vi "VALEW_ATC_Verify Concurrent.vi"(0 "GEA2 Reference In":refnum<k24>, 11 "Error In":errorcluster) -> (4 "GEA2 Reference Out":refnum<k24>, 6 "Pass/fail?":bool, 8 "Report Text":string, 15 "Error Out":errorcluster)   [LabVIEW 2016, in "TLMB.lvlib"]
doc: "This test covers the ATC algorithm when doing a concurrent fill. A concurrent fill allows both hot and cold valves to be on at the same time. The valves are operated in parallel."
uses:
  Projects/TLMB.lvlib
  Q:/Common/DLLs/GEA3/GeaCommunication.dll
  Common/DLLs/GEA3/GeaCommunication.dll
  Common/LabVIEW GEA2 Toolkit/LabVIEW_GEA2_Toolkit.lvlibp/type defs/Source_Destination.ctl
  TLMB Common/type defs/MC_Cycle_Engine_Request_State.ctl
  Common/LabVIEW GEA2 Toolkit/LabVIEW_GEA2_Toolkit.lvlibp/type defs/ERD Write Data In.ctl
  Common/LabVIEW GEA2 Toolkit/LabVIEW_GEA2_Toolkit.lvlibp/type defs/Data Type.ctl
  Common/LabVIEW GEA2 Toolkit/LabVIEW_GEA2_Toolkit.lvlibp/type defs/ERD Read Data In.ctl
  <vilib>/DAQmx/write.llb/DAQmx Write (Analog DBL 1Chan 1Samp).vi
  <vilib>/DAQmx/create/channels.llb/DAQmx Create Channel (AO-Voltage-Basic).vi
  <vilib>/DAQmx/miscellaneous.llb/DAQmx Fill In Error Info.vi
  Common/LabVIEW GEA2 Toolkit/LabVIEW_GEA2_Toolkit.lvlibp
panel:
  out "Valve time calculations pass?":bool
  out "Hot valve DAQ pass?":bool
  out "Cold valve DAQ pass?":bool
  out "Calc bath temp after seg gals":dbl
  out "Bath temp after seg gals":dbl
  out "Bath temp updated after segment fill?":bool
  in  "Standalone?":bool
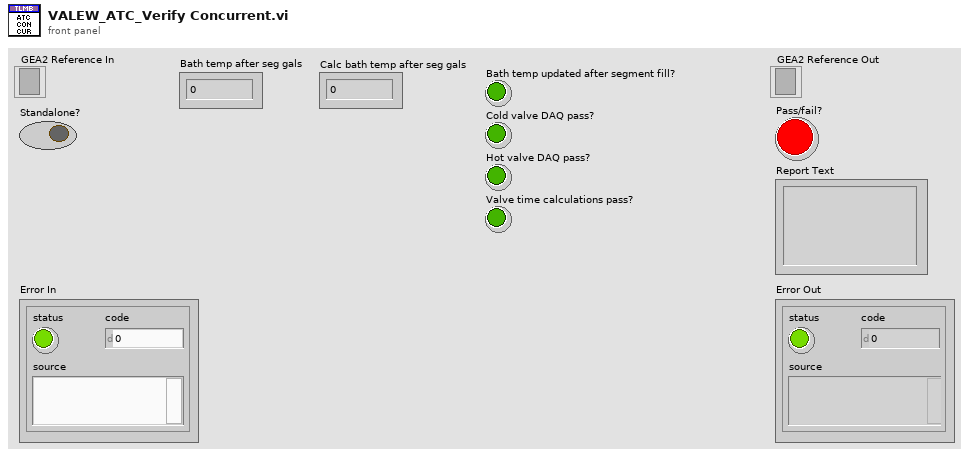
[diagram p1: front panel]
types:
  T1 = enum16{"EQ (==)", "NE (!=)", "GT (>)", "LT (<)", "GE (>=)", "LE (<=)", "GTLT(> <)", "GELE (>= <=)", "GELT (>= <)", "GTLE (> <=)", "LTGT (< >)", "LEGE (<= >=)", "LEGT (<= >)", "LTGE (< >=)", "No Comparison"}
  T2 = typedef "LabVIEW_GEA2_Toolkit.lvlibp/Source_Destination.ctl" = cluster{"Source":u8, "Destination":u8}
  T3 = typedef "TLMB.lvlib/MC_Cycle_Engine_Request_State.ctl" = enum16{"Select", "Start", "Pause", "Resume", "Stop"}
  T4 = typedef "LabVIEW_GEA2_Toolkit.lvlibp/ERD Read Data In.ctl" = cluster{"ERD Number":u16, "Data Type":T5}
  T5 = typedef "LabVIEW_GEA2_Toolkit.lvlibp/Data Type.ctl" = enum16{"string", "boolean", "uint8_t", "uint16_t", "uint32_t", "uint64_t", "int8_t", "int16_t", "int32_t", "int64_t"}
  T6 = typedef "LabVIEW_GEA2_Toolkit.lvlibp/ERD Write Data In.ctl" = cluster{"ERD Number":u16, "Data Type":T5, "Data":string}
  T7 = typedef "TLMB.lvlib/VALEW_ATC_Data.ctl" = cluster{"Accumulated hot gallons":dbl, "Accumulated cold gallons":dbl, "Current tub gallons":dbl, "Cold inlet temp (F)":dbl, "Hot inlet temp (F)":dbl, "Warm inlet temp (F)":dbl, "Hot valve time (s)":u16, "Cold valve time (s)":u16, "Current bath temp (F)":dbl, "Current water temp (F)":dbl, "Segment gallons":dbl}
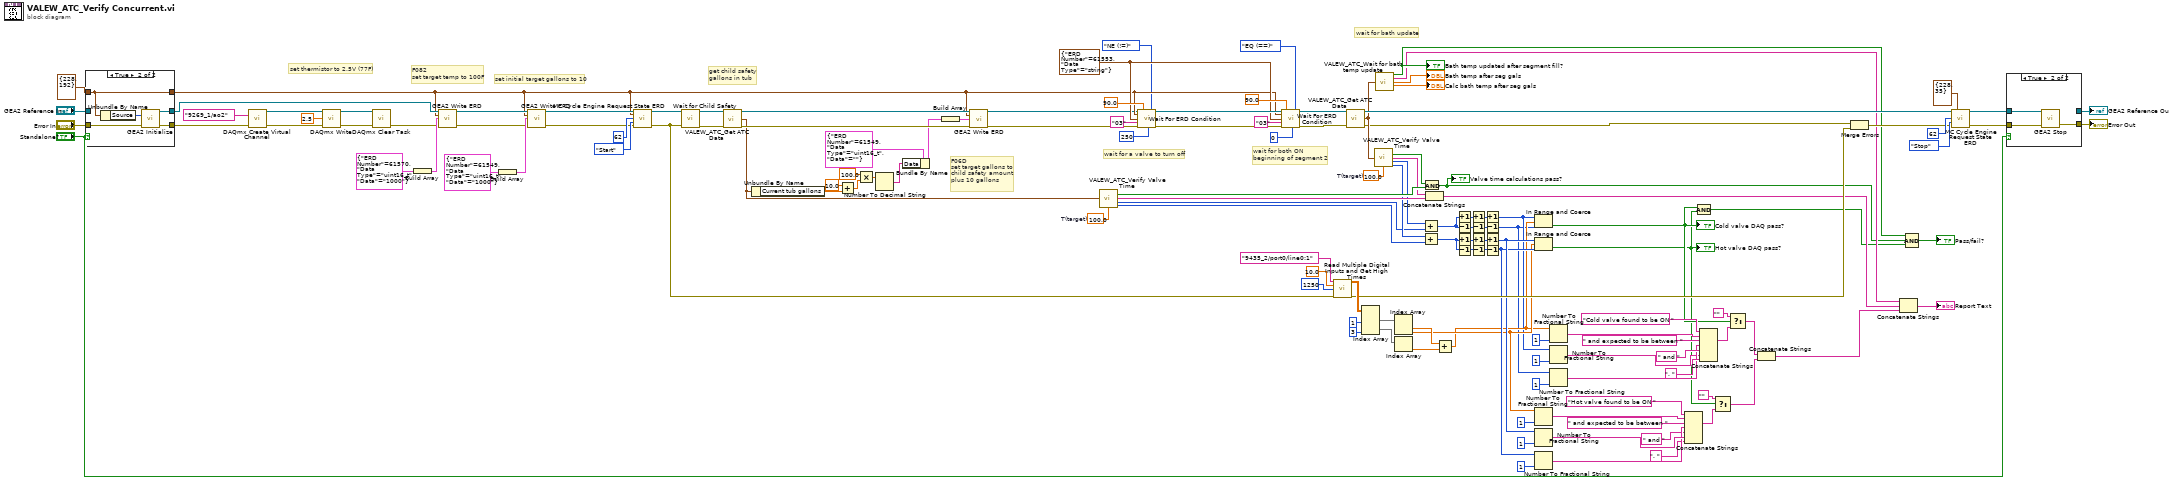
[diagram p0: block diagram]
diagram:
  w93 = 100.0  # T(target)
  w94 = 100.0  # T(target)
  w100 = T4 {"ERD Number"=61553, "Data Type"=enum."string"} ("ERD Read Data")
  # "set thermistor to 2.5V (77F)"
  # "wait for bath update"
  # "wait for both ON\nbeginning of segment 2"
  # "wait for a valve to turn off"
  # "set initial target gallons to 10"
  # "F06D\nset target gallons to\nchild safety amount\nplus 10 gallons"
  # "get child safety\ngallons in tub"
  # "F082\nset target temp to 100F"
  n1 = case shown="True" "Standalone?" {
    tunnel: T2 {"Source"=228, "Destination"=192} ("GEA Inputs") -> [w141 w144]
    tunnel: [w143 w147] -> w127
    tunnel: [w142 w146] -> w71
    tunnel: "Error In" -> [w142 w145]
    tunnel: "GEA2 Reference In" -> [w143 _]
    tunnel: [w141 w144] -> w68
    frame False {
    }
    frame True {
      n2 = Unbundle By Name(w144) -> ("Source"=w148:u8)
      n3 = call "GEA2 Initialize.vi"("Source Address"=w148, "error in"=w145) -> ("GEA2 Reference Out"=w147:refnum<k24>, "error out"=w146:errorcluster)  [unwired: 11 in, 1 out]
    }
  }
  n4 = call-poly <vilib>:"DAQmx Create Virtual Channel.vi"("physical channels"=tag "9269_1/ao2", "error in"=w71) -> ("task out"=w76:refnum<k21>, "error out"=w70:errorcluster)  [unwired: 12 in]
  n5 = call-poly <vilib>:"DAQmx Write.vi"("task/channels in"=w76, "data"=2.5, "error in"=w70) -> ("task out"=w72:refnum<k21>, "error out"=w73:errorcluster)  [unwired: 10 in, 1 out]
  n6 = call <vilib>:"DAQmx Clear Task.vi"("task in"=w72, "error in"=w73) -> ("error out"=w69:errorcluster)  [unwired: 13 in]
  n7 = Build Array(T6 {"ERD Number"=61570, "Data Type"=enum."uint16_t", "Data"="1000"} ("ERD Write Data In")) -> (w134:T6[])
  n8 = call "GEA2 Write ERD.vi"("GEA2 Reference In"=w127, "GEA Inputs"=w68, "Write ERD List"=w134, "Error In"=w69) -> ("GEA2 Reference Out"=w116:refnum<k24>, "Error Out"=w115:errorcluster)  [unwired: 9 in, 1 out]
  n9 = Build Array(T6 {"ERD Number"=61549, "Data Type"=enum."uint16_t", "Data"="1000"} ("ERD Write Data In")) -> (w117:T6[])
  n10 = call "GEA2 Write ERD.vi"("GEA2 Reference In"=w116, "GEA Inputs"=w68, "Write ERD List"=w117, "Error In"=w115) -> ("GEA2 Reference Out"=w114:refnum<k24>, "Error Out"=w113:errorcluster)  [unwired: 9 in, 1 out]
  n11 = call "MC Cycle Engine Request State ERD.vi"("GEA2 Reference In"=w114, "GEA Inputs"=w68, "Cycle #"=u8 62, "MC Cycle Engine State"=MC_Cycle_Engine_Request_State."Start", "Error In"=w113) -> ("GEA2 Reference Out"=w136:refnum<k24>, "Error Out"=w66:errorcluster)  [unwired: 9 in]
  n12 = call "Wait for Child Safety.vi"("GEA2 Reference In"=w136, "Error In"=w66) -> ("GEA2 Reference Out"=w88:refnum<k24>, "Error Out"=w81:errorcluster)  [unwired: 9 in, 3 out]
  n13 = call "VALEW_ATC_Get ATC Data.vi"("GEA2 Reference In"=w88, "Error In"=w81) -> ("GEA2 Reference Out"=w125:refnum<k24>, "ATC Data"=w3:T7, "Error Out"=w126:errorcluster)  [unwired: 11 in]
  n14 = Unbundle By Name(w3) -> ("Current tub gallons"=w99:dbl)
  n15 = Add(x=10.0, y=w99) -> (x+y=w120:dbl)
  n16 = Multiply(x=100.0, y=w120) -> (x*y=w121:dbl)
  n17 = Number To Decimal String(number=w121) -> (decimal integer string=w112:string)  [unwired: 1 in]
  n18 = Bundle By Name(cluster=T6 {"ERD Number"=61549, "Data Type"=enum."uint16_t", "Data"=""} ("ERD Write Data In"), "Data"=w112) -> (w122:T6)
  n19 = Build Array(w122) -> (w133:T6[])
  n20 = call "GEA2 Write ERD.vi"("GEA2 Reference In"=w125, "GEA Inputs"=w68, "Write ERD List"=w133, "Error In"=w126) -> ("GEA2 Reference Out"=w1:refnum<k24>, "Error Out"=w2:errorcluster)  [unwired: 9 in, 1 out]
  n21 = call "VALEW_ATC_Verify Valve Time.vi"("ATC Data"=w3, "T(target)"=w94) -> ("Pass/Fail?"=w91:bool, "Report Text"=w89:string, "Cold valve time (s) ATC"=w78:u16, "Hot valve time (s) ATC"=w77:u16)  [unwired: 10 in]
  n22 = call "Wait For ERD Condition.vi"("GEA2 Reference In"=w1, "GEA Inputs"=w68, "ERD Read Data"=w100, "Expected Low"="03", "Error In"=w2, "Timeout (s)"=90.0, "Loop Rate (ms)"=u32 250, "Comparison"=T1."NE (!=)") -> ("GEA2 Reference Out"=w111:refnum<k24>, "Error Out"=w110:errorcluster)  [unwired: 7 in, 3 out]
  n23 = call "Wait For ERD Condition.vi"("GEA2 Reference In"=w111, "GEA Inputs"=w68, "ERD Read Data"=w100, "Expected Low"="03", "Error In"=w110, "Timeout (s)"=90.0, "Loop Rate (ms)"=u32 0, "Comparison"=T1."EQ (==)") -> ("GEA2 Reference Out"=w96:refnum<k24>, "Error Out"=w97:errorcluster)  [unwired: 7 in, 3 out]
  n24 = call "Read Multiple Digital Inputs and Get High Times.vi"("Lines"=tag "9435_2/port0/line0:1", "Rate (Hz)"=10.0 ("rate"), "Samples"=1250 ("samples per channel"), "Error In"=w66) -> ("High Times (s)"=w84:dbl[][], "Error Out"=w49:errorcluster)  [unwired: 10 in]
  n25 = call "VALEW_ATC_Get ATC Data.vi"("GEA2 Reference In"=w96, "Error In"=w97) -> ("GEA2 Reference Out"=w98:refnum<k24>, "ATC Data"=w67:T7, "Error Out"=w48:errorcluster)  [unwired: 11 in]
  n26 = Index Array(array=w84, index (col) #1=1 ("disabled index (col)"), index (col) #2=3 ("index (col)")) -> (element #1=w82:dbl[], element #2=w55:dbl[])  [unwired: 2 in]
  n27 = call "VALEW_ATC_Verify Valve Time.vi"("ATC Data"=w67, "T(target)"=w93) -> ("Pass/Fail?"=w92:bool, "Report Text"=w90:string, "Cold valve time (s) ATC"=w80:u16, "Hot valve time (s) ATC"=w79:u16)  [unwired: 10 in]
  n28 = call "VALEW_ATC_Wait for bath temp update.vi"("ATC Data"=w67) -> ("Bath temp updated after segment fill?"=w46:bool, "Report Text"=w43:string, "Bath temp after seg gals"=→"Bath temp after seg gals":dbl, "Calc bath temp after seg gals"=→"Calc bath temp after seg gals":dbl)  [unwired: 11 in]
  "Bath temp updated after segment fill?" <- w46
  n29 = Index Array(array=w82) -> (element #1=w53:dbl, element #2=w28:dbl)  [unwired: 2 in]
  n30 = Index Array(array=w55) -> (element=w54:dbl)  [unwired: 1 in]
  n31 = Add(x=w80, y=w78) -> (x+y=w58:u16)
  n32 = Add(x=w79, y=w77) -> (x+y=w57:u16)
  n33 = And(x=w92, y=w91) -> (x .and. y?=w8:bool)
  "Valve time calculations pass?" <- w8
  n34 = Concatenate Strings(w90, w89) -> (w7:string)
  n35 = Add(x=w53, y=w54) -> (x+y=w15:dbl)
  n36 = Increment(x=w58) -> (x+1=w62:u16)
  n37 = Decrement(x=w58) -> (x-1=w65:u16)
  n38 = Increment(x=w57) -> (x+1=w64:u16)
  n39 = Decrement(x=w57) -> (x-1=w63:u16)
  n40 = Increment(x=w62) -> ()  [unwired: 1 out]
  n41 = Decrement(x=w65) -> (x-1=w61:u16)
  n42 = Increment(x=w64) -> (x+1=w60:u16)
  n43 = Decrement(x=w63) -> (x-1=w59:u16)
  n44 = Increment(x=w62) -> (x+1=w14:u16)
  n45 = Decrement(x=w61) -> (x-1=w13:u16)
  n46 = Increment(x=w60) -> (x+1=w31:u16)
  n47 = Decrement(x=w59) -> (x-1=w30:u16)
  n48 = In Range and Coerce(upper limit=w14, x=w15, lower limit=w13) -> (In Range?=w10:bool)  [unwired: 1 out]
  "Cold valve DAQ pass?" <- w10
  n49 = In Range and Coerce(upper limit=w31, x=w28, lower limit=w30) -> (In Range?=w9:bool)  [unwired: 1 out]
  "Hot valve DAQ pass?" <- w9
  n50 = Number To Fractional String(number=w28, precision (6)=i16 1) -> (F-format string=w37:string)  [unwired: 2 in]
  n51 = Number To Fractional String(number=w31, precision (6)=i16 1) -> (F-format string=w42:string)  [unwired: 2 in]
  n52 = Number To Fractional String(number=w30, precision (6)=i16 1) -> (F-format string=w35:string)  [unwired: 2 in]
  n53 = Number To Fractional String(number=w15, precision (6)=i16 1) -> (F-format string=w21:string)  [unwired: 2 in]
  n54 = Number To Fractional String(number=w14, precision (6)=i16 1) -> (F-format string=w16:string)  [unwired: 2 in]
  n55 = Number To Fractional String(number=w13, precision (6)=i16 1) -> (F-format string=w23:string)  [unwired: 2 in]
  n56 = Concatenate Strings("Hot valve found to be ON ", w37, " and expected to be between ", w35, " and " ("string"), w42, ". " ("string")) -> (w32:string)
  n57 = Compound Arithmetic op=AND(w10, w9) -> (w6:bool)
  n58 = Concatenate Strings("Cold valve found to be ON ", w21, " and expected to be between ", w23, " and " ("string"), w16, ". " ("string")) -> (w26:string)
  n59 = Select(t="", s=w9, f=w32) -> (s? t:f=w11:string)
  n60 = Select(t="", s=w10, f=w26) -> (s? t:f=w12:string)
  n61 = Concatenate Strings(w12, w11) -> (w5:string)
  n62 = Merge Errors(w48, w49) -> (w47:errorcluster)
  n63 = Concatenate Strings(w43, w7, w5) -> (→"Report Text":string)
  n64 = Compound Arithmetic op=AND(w46, w8, w6) -> (→"Pass/fail?":bool)
  n65 = call "MC Cycle Engine Request State ERD.vi"("GEA2 Reference In"=w98, "GEA Inputs"=T2 {"Source"=228, "Destination"=35}, "Cycle #"=u8 62, "MC Cycle Engine State"=MC_Cycle_Engine_Request_State."Stop", "Error In"=w47) -> ("GEA2 Reference Out"=w128:refnum<k24>, "Error Out"=w129:errorcluster)  [unwired: 9 in]
  n66 = case shown="True" "Standalone?" {
    tunnel: w129 -> [w150 w153]
    tunnel: w128 -> [w149 w152]
    tunnel: [w150 w151] -> w131
    tunnel: [w149 _] -> w132
    frame False {
    }
    frame True {
      n67 = call "GEA2 Stop.vi"("GEA2 Reference In"=w152, "Error In"=w153) -> ("Error Out"=w151:errorcluster)  [unwired: 13 in]
    }
  }
  "GEA2 Reference Out" <- w132
  "Error Out" <- w131
